vi "Projeto Termopar.vi"() -> ()   [LabVIEW 2020]
uses:
  <vilib>/express/express shared/transition.llb/Dynamic To Waveform Array.vi
  <vilib>/express/express signal manip/GetorSetDDTAttributes/Set DDT Attributes/SetT0.vi
  <vilib>/express/express shared/transition.llb/Waveform Array To Dynamic.vi
  <vilib>/express/express signal manip/GetorSetDDTAttributes/Set DDT Attributes/Set DDT Properties.xnode
panel:
  out "Saving Data 2":bool caption="Saving Data"
  out "Filename Out 2":path caption="Filename Out"
  in  "Filename 2":path=path "C:/Users/up201907151/Desktop/teste.xlsx" caption="Filename"
  out "Saving Data":bool
  out "Filename Out":path
  in  "Filename":path=path "C:/Users/up201907151/Desktop/teste.xlsx"
  in  "Enable":bool=TRUE
  out "Temp Termo vs calc":cluster{"Y":dbl[], "Y":dbl[]}[](graph) caption="XY Graph"
  out "T(ºC) Calc":dbl
  out "Vout":dbl
  out "Temperatura ºC":dbl
  out "Temp Termopar Tensao":cluster{"Y":dbl[], "Y":dbl[]}[](graph) caption="XY Graph"
  in  "stop":bool
  out "Waveform graph":dynamicdata(graph)
  out "data":dynamicdata(graph)
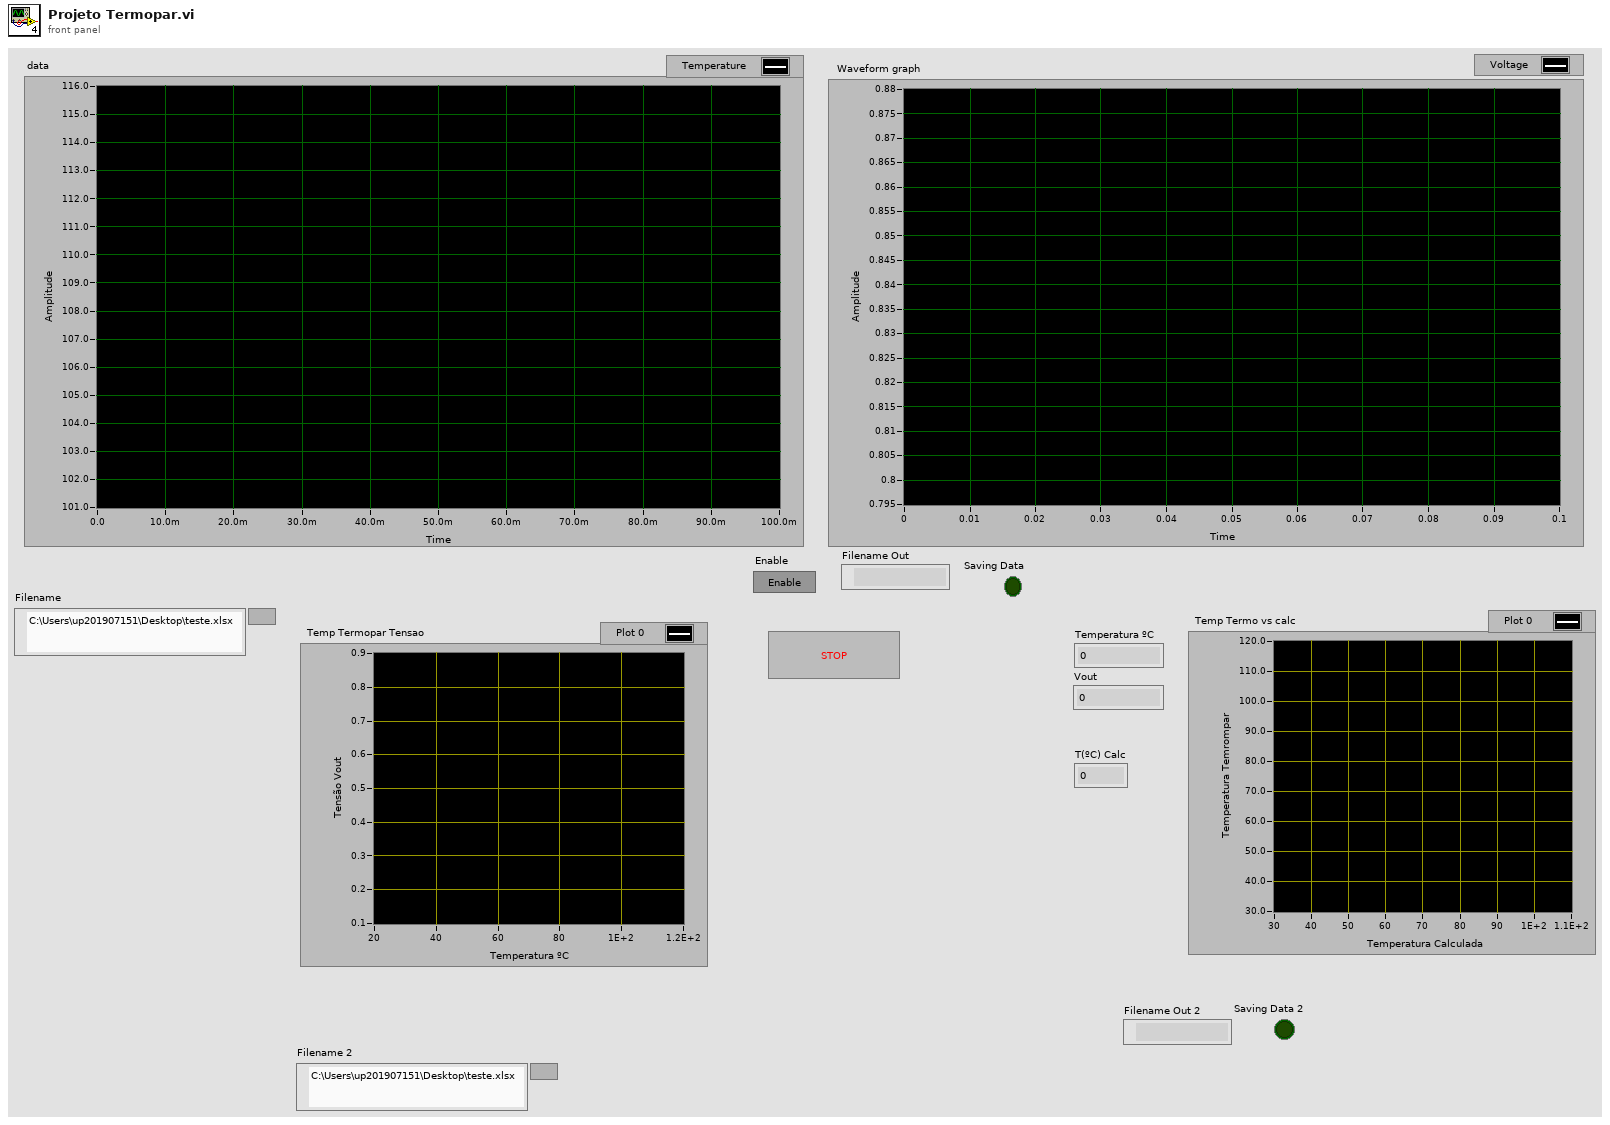
[diagram p1: front panel]
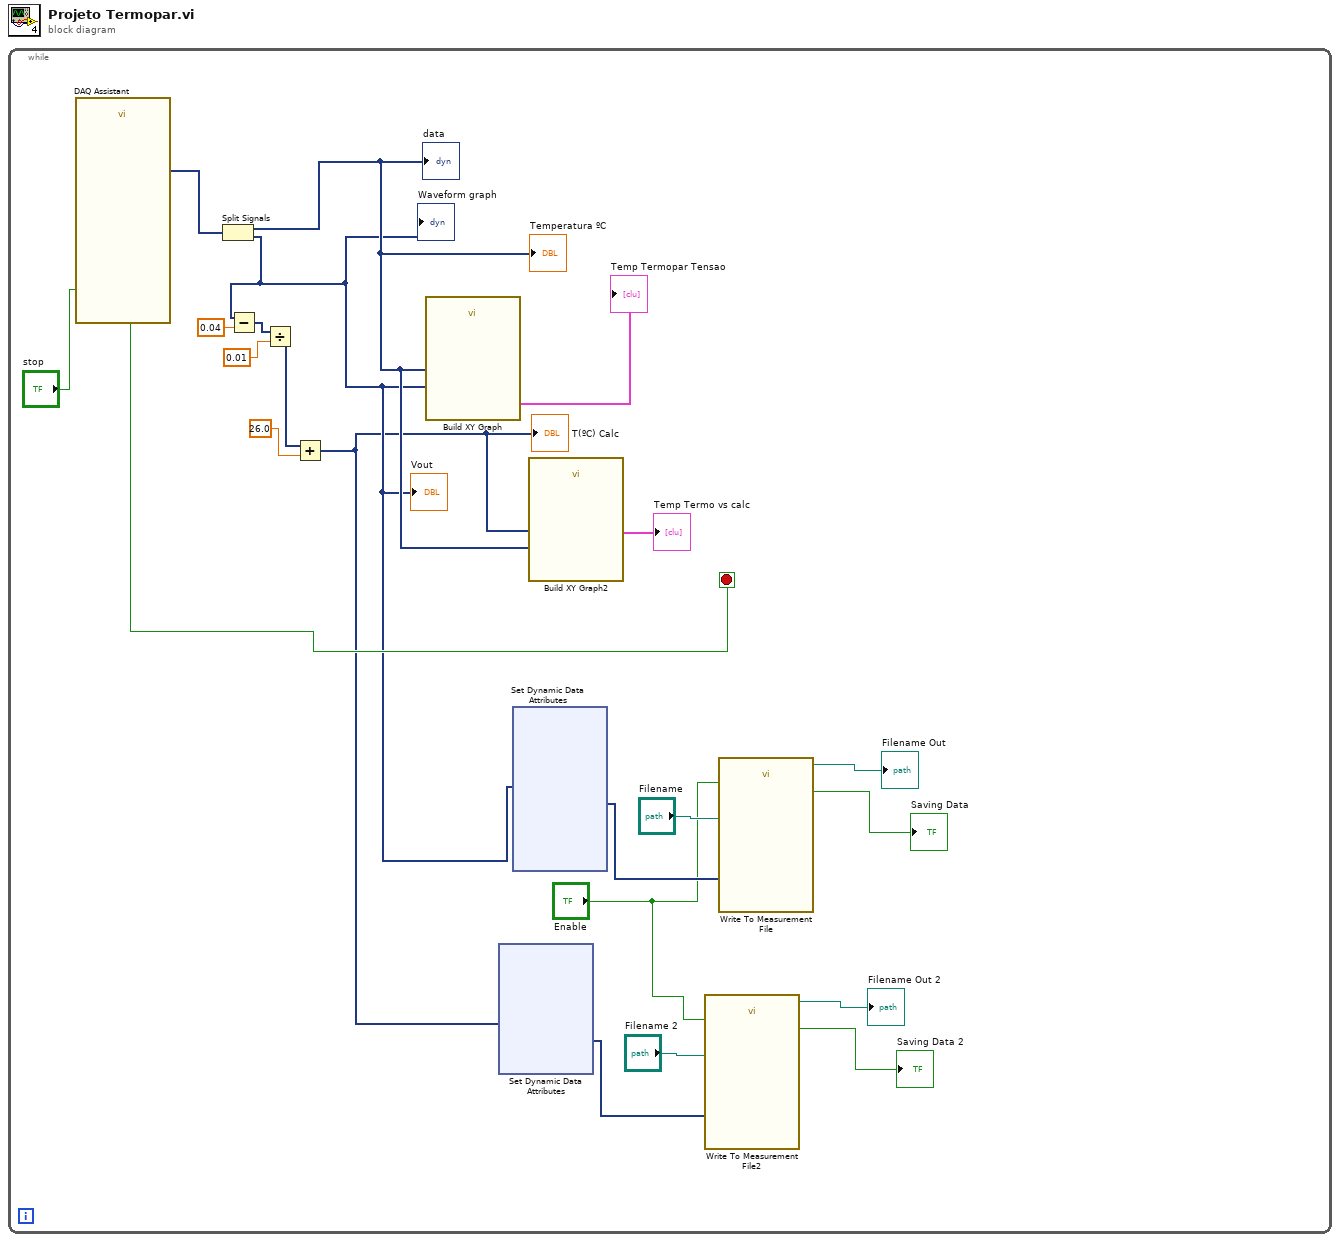
[diagram p0: block diagram]
diagram:
  n1 = while {
    stop <- w22 stop-if-true
    n2 = call "DAQ Assistant"("stop (F)"="stop") -> ("data"=w19:dynamicdata, "stopped"=w22:bool)  [unwired: 15 in, 2 out]
    n3 = Split Signals(w19) -> (w12:dynamicdata, w3:dynamicdata)  [unwired: 2 in]
    "data" <- w12
    "Waveform graph" <- w3
    "Temperatura ºC" <- w12
    "Vout" <- w3
    n4 = Subtract(x=w3, y=0.04) -> (x-y=w14:dynamicdata)
    n5 = Divide(x=w14, y=0.01) -> (x/y=w17:dynamicdata)
    n6 = Add(x=w17, y=26.0) -> (x+y=w2:dynamicdata)
    "T(ºC) Calc" <- w2
    n7 = call "Build XY Graph"("Y Input"=w3, "X Input"=w12) -> ("XY Graph"=→"Temp Termopar Tensao":cluster{"X":dbl[], "Y":dbl[]}[])  [unwired: 8 in, 1 out]
    n8 = xnode "Set Dynamic Data Attributes"("Signals In"=w2) -> ("Signals Out"=w7:dynamicdata)  [unwired: 2 in, 1 out]
    n9 = xnode "Set Dynamic Data Attributes"("Signals In"=w3) -> ("Signals Out"=w11:dynamicdata)  [unwired: 2 in, 1 out]
    n10 = call "Build XY Graph2"("Y Input"=w12, "X Input"=w2) -> ("XY Graph"=→"Temp Termo vs calc":cluster{"X":dbl[], "Y":dbl[]}[])  [unwired: 8 in, 1 out]
    n11 = call "Write To Measurement File2"("Signals"=w7, "Enable"="Enable", "Filename"="Filename 2") -> ("Filename Out"=→"Filename Out 2":path, "Saving Data"=→"Saving Data 2":bool)  [unwired: 14 in, 1 out]
    n12 = call "Write To Measurement File"("Signals"=w11, "Enable"="Enable", "Filename"="Filename") -> ("Filename Out"=→"Filename Out":path, "Saving Data"=→"Saving Data":bool)  [unwired: 14 in, 1 out]
  }
